vi "Reset Input Protection.vi"(8 "error in (no error)":errorcluster, 11 "VISA resource name":refnum<visa-resource-name>) -> (0 "error out":errorcluster, 3 "VISA resource name out":refnum<visa-resource-name>)   [LabVIEW 2018, in "BK Precision 8600 Series.lvlib"]
doc: "Resets the status of over power protection (OPP) and over current protection (OCP).\n\nNote: If input state was ON/ENABLED prior to the protection trip, resetting the protection will not disable the input, allowing it to run in its previous settings. This in turn may allow the load to trip the protection again under the same settings if OPP and/or OCP conditions are met. It is recommended to disable the input state using <b>Enable Inputs.vi</b> immediatelyh after running this vi to verify the instrument's settings or load condition."
uses:
  <instrlib>/BK Precision 8600 Series/BK Precision 8600 Series.lvlib
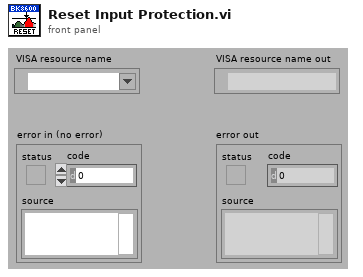
[diagram p1: front panel]
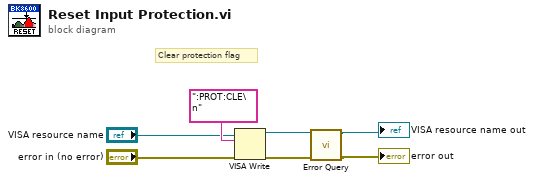
[diagram p0: block diagram]
diagram:
  # "Clear protection flag"
  n1 = VISA Write(VISA resource name="VISA resource name", write buffer=":PROT:CLE\n", error in (no error)="error in (no error)") -> (VISA resource name out=w4:refnum<visa-resource-name>, error out=w3:errorcluster)  [unwired: 1 out]
  n2 = call <instrlib>:"Error Query.vi"("error in (no error)"=w3, "VISA resource name"=w4) -> ("error out"=→"error out":errorcluster, "VISA resource name out"=→"VISA resource name out":refnum<visa-resource-name>)  [unwired: 6 in, 2 out]
